vi "Configure External Device Flag.vi"(8 "error in (no error)":errorcluster, 9 "on":bool, 10 "flag index":u8, 11 "Lotis in":refnum<class "PL Lotis TII LS.lvclass">) -> (0 "error out":errorcluster, 3 "Lotis out":refnum<class "PL Lotis TII LS.lvclass">)   [LabVIEW 2015, in "PL Lotis TII LS.lvclass"]
doc: "Configures external device flag."
uses:
  PL Lotis TII LS.lvclass
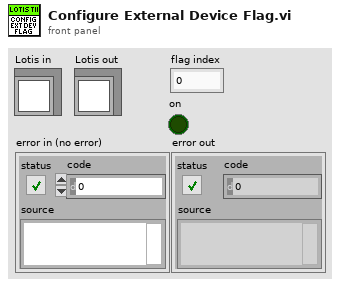
[diagram p1: front panel]
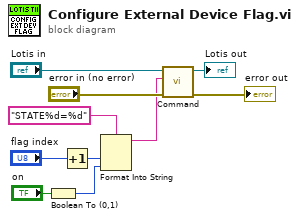
[diagram p0: block diagram]
diagram:
  n1 = Boolean To (0,1)(Boolean="on") -> (0, 1=w1:i16)
  n2 = Increment(x="flag index") -> (x+1=w3:u8)
  n3 = Format Into String(format string="STATE%d=%d" ("command"), w3, w1) -> (resulting string=w4:string)  [unwired: 2 in, 1 out]
  n4 = call "Command.vi"("error in (no error)"="error in (no error)", "command"=w4, "Lotis in"="Lotis in") -> ("error out"=→"error out":errorcluster, "Lotis out"=→"Lotis out":refnum<class "PL Lotis TII LS.lvclass">)  [unwired: 6 in, 1 out]
